vi "programa 7.vi"() -> ()   [LabVIEW 2011]
panel:
  in  "Salir":bool
  in  "Suma mas":bool
  out "Menor":dbl
  out "Mayor":dbl
  out "Promedio":dbl
  out "Suma":dbl
  out "Array":dbl[](array[numeric])
  in  "Generar":bool
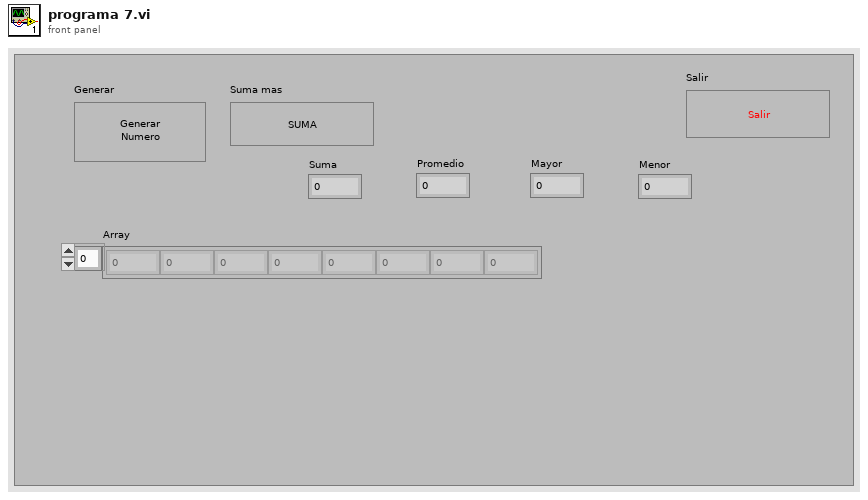
[diagram p1: front panel]
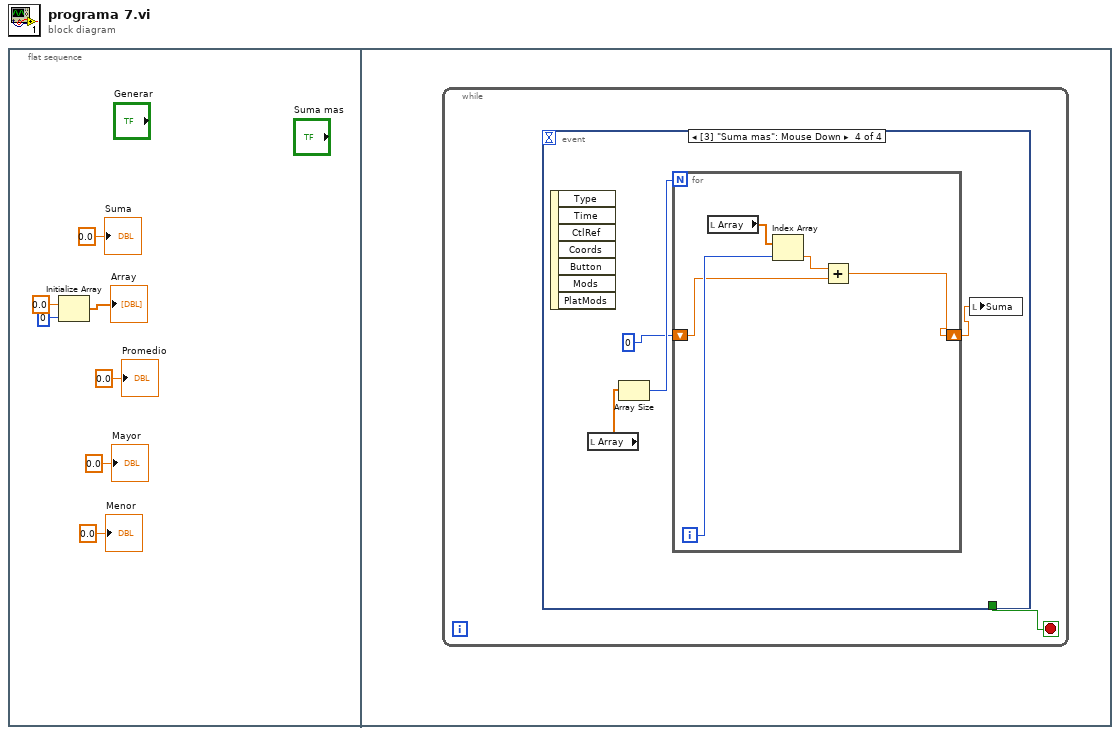
[diagram p0: block diagram]
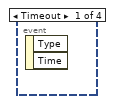
[diagram p2: hidden frame]
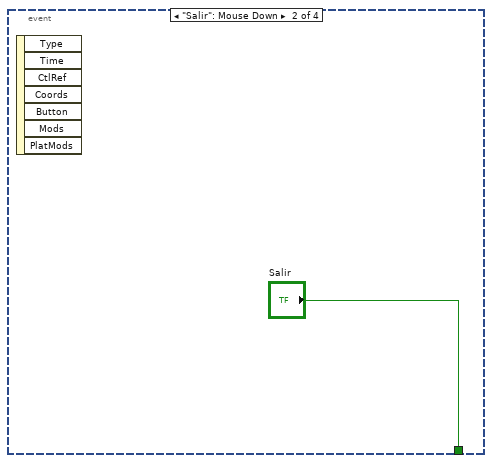
[diagram p3: hidden frame]
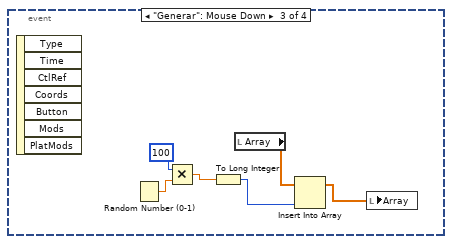
[diagram p4: hidden frame]
diagram:
  n1 = flat-sequence {
    frame #0 {
      n2 = Initialize Array(0.0 ("element"), 0 ("dimension size")) -> (→"Array":dbl[])
      "Suma" <- 0.0 ("Suma")
      "Promedio" <- 0.0 ("Promedio")
      "Mayor" <- 0.0 ("Mayor")
      "Menor" <- 0.0 ("Menor")
    }
    frame #1 {
      n3 = while {
        stop <- w8 stop-if-true
        n4 = event shown="[3] \"Suma mas\": Mouse Down" {
          selector: _ -> [_ _ _ _]
          dyn-events: _ -> [_ _ _ _]
          timeout: _ -> [_ _ _ _]
          tunnel: [_ "Salir" _ _] -> w8
          event Timeout {
            n5 = event-data() -> ()  [unwired: 1 in, 2 out]
          }
          event "Salir": Mouse Down {
            n6 = event-data() -> ()  [unwired: 1 in, 7 out]
          }
          event "Generar": Mouse Down {
            n7 = event-data() -> ()  [unwired: 1 in, 7 out]
            n8 = Random Number (0-1)() -> (number: 0 to 1=w14:dbl)
            n9 = Multiply(x=100, y=w14) -> (x*y=w13:dbl)
            n10 = To Long Integer(number=w13) -> (32bit integer=w12:i32)
            n11 = local read "Array"() -> (w11:dbl[])
            n12 = Insert Into Array(array=w11, new element=w12) -> (w10:dbl[])  [unwired: 1 in]
            n13 = local write "Array"(w10) -> ()
          }
          event "Suma mas": Mouse Down {
            n14 = event-data() -> ()  [unwired: 1 in, 7 out]
            n15 = local read "Array"() -> (w19:dbl[])
            n16 = Array Size(array=w19) -> (size(s)=w18:i32)
            n17 = for {
              N: w18 -> [_]
              shift-right: [w20] -> w16
              shift-left: 0 -> [w21]
              i -> [w23]
              n18 = local read "Array"() -> (w24:dbl[])
              n19 = Index Array(array=w24, index=w23) -> (element=w22:dbl)
              n20 = Add(x=w22, y=w21) -> (x+y=w20:dbl)
            }
            n21 = local write "Suma"(w16) -> ()
          }
        }
      }
    }
  }
